vi "_RT_Pub getEnumString.vi"(1 "system type":T1) -> (0 "element":string)   [LabVIEW 2018]
uses:
  Ctl/_ctl_RT_SysLog.ctl
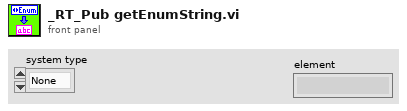
[diagram p1: front panel]
types:
  T1 = typedef "_ctl_RT_SysLog.ctl" = enum16{"None", "Initialize", "StartupRT", "StartupFPGA", "StartupAllocator", "GetMass", "SetWfmCode", "SetLaserCtrl", "SetTurboCtrl", "SetD999Ctrl", "Reconnecting...", "Interrupt", "StopRT"}
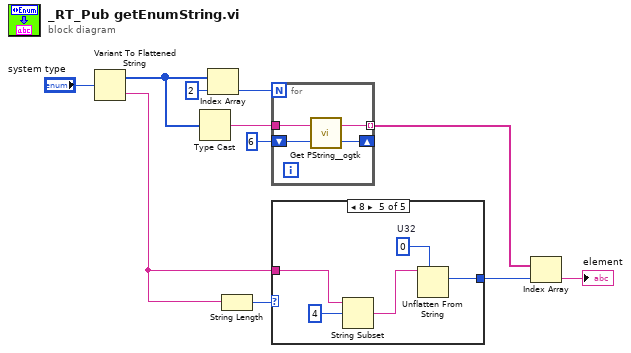
[diagram p0: block diagram]
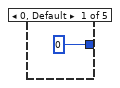
[diagram p2: hidden frame]
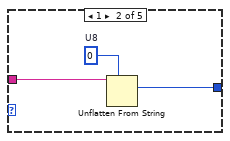
[diagram p3: hidden frame]
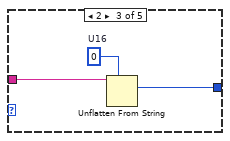
[diagram p4: hidden frame]
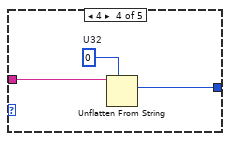
[diagram p5: hidden frame]
diagram:
  n1 = Variant To Flattened String(Variant="system type") -> (data string=w3:string, 1:w7:i16[])
  n2 = Type Cast(x=w7) -> (*(type *) &x=w1:string)  [unwired: 1 in]
  n3 = Index Array(array=w7, index=2) -> (element=w9:i16)
  n4 = String Length(string=w3) -> (length=w4:i32)
  n5 = for {
    N: w9 -> [_]
    shift-right: [w13] -> _
    shift-left: 6 -> [w14]
    tunnel: [w15] -> w6 mode=indexing
    tunnel: w1 -> [w12]
    n6 = call <userlib>:"Get PString__ogtk.vi"("offset (0)"=w14, "String"=w12) -> ("offset past PString"=w13:i32, "PString"=w15:string)
  }
  n7 = case shown="8" w4 {
    tunnel: w3 -> [_ w19 w22 w25 w27]
    tunnel: [u32 0 ("U32") w18 w21 w24 w30] -> w2
    frame 0, Default {
    }
    frame 1 {
      w17 = u8 0  # U8
      n8 = Unflatten From String(type=w17, binary string=w19) -> (value=w18:u8)  [unwired: 3 in, 2 out]
    }
    frame 2 {
      w20 = u16 0  # U16
      n9 = Unflatten From String(type=w20, binary string=w22) -> (value=w21:u16)  [unwired: 3 in, 2 out]
    }
    frame 4 {
      w23 = u32 0  # U32
      n10 = Unflatten From String(type=w23, binary string=w25) -> (value=w24:u32)  [unwired: 3 in, 2 out]
    }
    frame 8 {
      w26 = u32 0  # U32
      n11 = String Subset(string=w27, offset (0)=4) -> (substring=w28:string)  [unwired: 1 in]
      n12 = Unflatten From String(type=w26, binary string=w28) -> (value=w30:u32)  [unwired: 3 in, 2 out]
    }
  }
  n13 = Index Array(array=w6, index=w2) -> (element=→"element":string)
